vi "GenerateTriggerPulse.vi"(2 "Trigger":bool=TRUE, 3 "Pulse Width [cycles]":u16) -> (0 "Out":bool, 1 "Count out":u16)   [LabVIEW 2020]
uses:
  <instrlib>/_niInstr/Basic Elements/v1/FPGA/Private/Count Up U16.vi
  <instrlib>/_niInstr/Basic Elements/v1/FPGA/niInstr Basic Elements v1 FPGA.lvlib
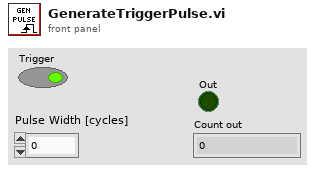
[diagram p1: front panel]
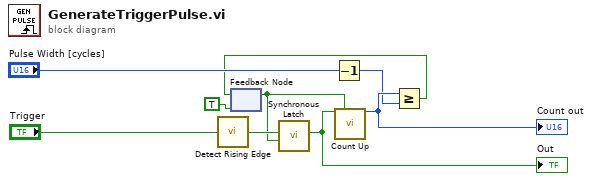
[diagram p0: block diagram]
diagram:
  n1 = call <instrlib>:"Detect Rising Edge.vi"("signal"="Trigger") -> ("edge detected"=w4:bool)  [unwired: 14 in]
  n2 = feedback #1(TRUE) -> (w2:bool)
  n3 = call <instrlib>:"Synchronous Latch.vi"("clear"=w2, "set"=w4) -> ("out"=w1:bool)  [unwired: 9 in]
  "Out" <- w1
  n4 = Decrement(x="Pulse Width [cycles]") -> (x-1=w8:u16)
  n5 = call-poly <instrlib>:"Count Up.vi"("increment"=w1, "reset"=w2) -> ("count out"=w9:u16)  [unwired: 13 in]
  "Count out" <- w9
  n6 = Greater Or Equal?(x=w9, y=w8) -> (x >= y?=w6:bool)
  n7 = feedback-in #1(w6) -> ()
